vi "ReadSudoku.vi"(11 "Jpeg path":path) -> (0 "error out":errorcluster, 2 "image data":T1, 3 "Picture":picture)   [LabVIEW 2020]
uses:
  <vilib>/picture/picture.llb/imagedata.ctl
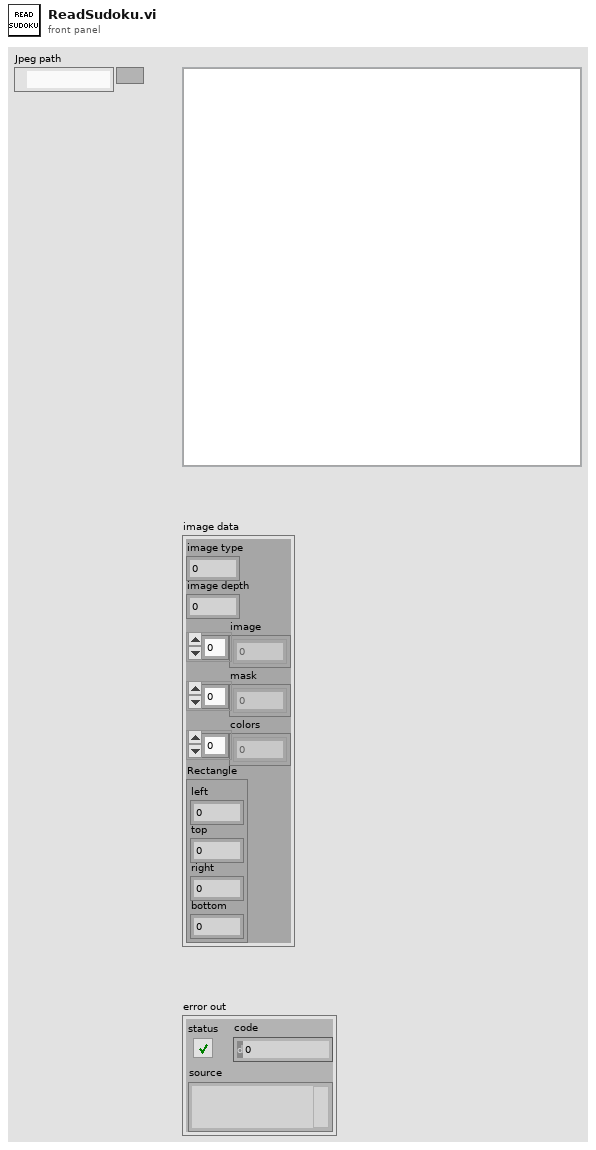
[diagram p1: front panel]
types:
  T1 = typedef "imagedata.ctl" = cluster{"image type":i32, "image depth":i32, "image":u8[], "mask":u8[], "colors":u32[], "Rectangle":cluster{"left":i16, "top":i16, "right":i16, "bottom":i16}}
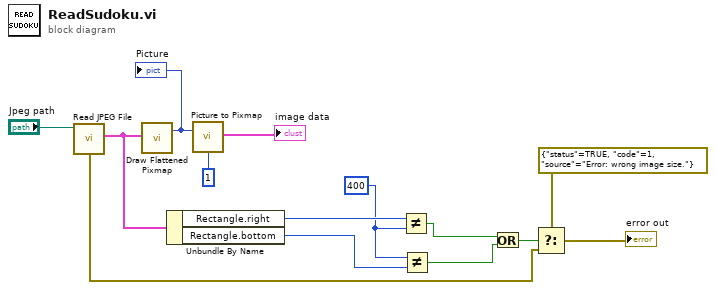
[diagram p0: block diagram]
diagram:
  w7 = 400
  n1 = call <vilib>:"Read JPEG File.vi"("path to JPEG file"="Jpeg path") -> ("error out"=w3:errorcluster, "image data"=w10:T1)  [unwired: 8 in, 1 out]
  n2 = call <vilib>:"Draw Flattened Pixmap.vi"("image data"=w10) -> ("new picture"=w14:picture)  [unwired: 8 in]
  "Picture" <- w14
  n3 = Unbundle By Name(w10) -> ("Rectangle.right"=w9:i16, "Rectangle.bottom"=w8:i16)
  n4 = call <vilib>:"Picture to Pixmap.vi"("depth"=1, "picture"=w14) -> ("image data"=→"image data":T1)  [unwired: 8 in, 1 out]
  n5 = Not Equal?(x=w9, y=w7) -> (x != y?=w6:bool)
  n6 = Not Equal?(x=w7, y=w8) -> (x != y?=w5:bool)
  n7 = Or(x=w6, y=w5) -> (x .or. y?=w4:bool)
  n8 = Select(t=errorcluster {"status"=TRUE, "code"=1, "source"="Error: wrong image size."}, s=w4, f=w3) -> (s? t:f=→"error out":errorcluster)
